vi "BuildingSingleImageGreyLevelDataBase.vi"(6 "Running Index":i32, 8 "error in (no error)":errorcluster, 9 "ConfDB":T1={"NumberOfImages"=0, "NoImages2SaveAroundFreeze"=0, "Path"=path "", "NameOfPartialFile"="", "StartIndex"=0, "NumberOfStdTol"=0, "Detla t (sec)"=2, "Number of images for baseline"=10, "Temperature File Name"="", "Score"=15.0, "Index number of Files"=[], "End Index"=2187, "Temperature Array"=[], "TStartIndex"=2187}, 10 "Droplet Bounding Box":cluster{"x":sgl, "y":sgl}[][](array[cluster]), 11 "Image Ref In":T2) -> (0 "error out":errorcluster, 1 "Difference in Grey Level":dbl[](array[numeric]), 2 "GreyLevelArray":dbl[](array[numeric]))   [LabVIEW 2013]
doc: "Go over all images and retrieve Grey level of each drop and the difference between the i+1 and i image"
uses:
  <vilib>/vision/Image Controls.llb/IMAQ Image.ctl
  DB/ConfDB.ctl
  DB/DbEnum.ctl
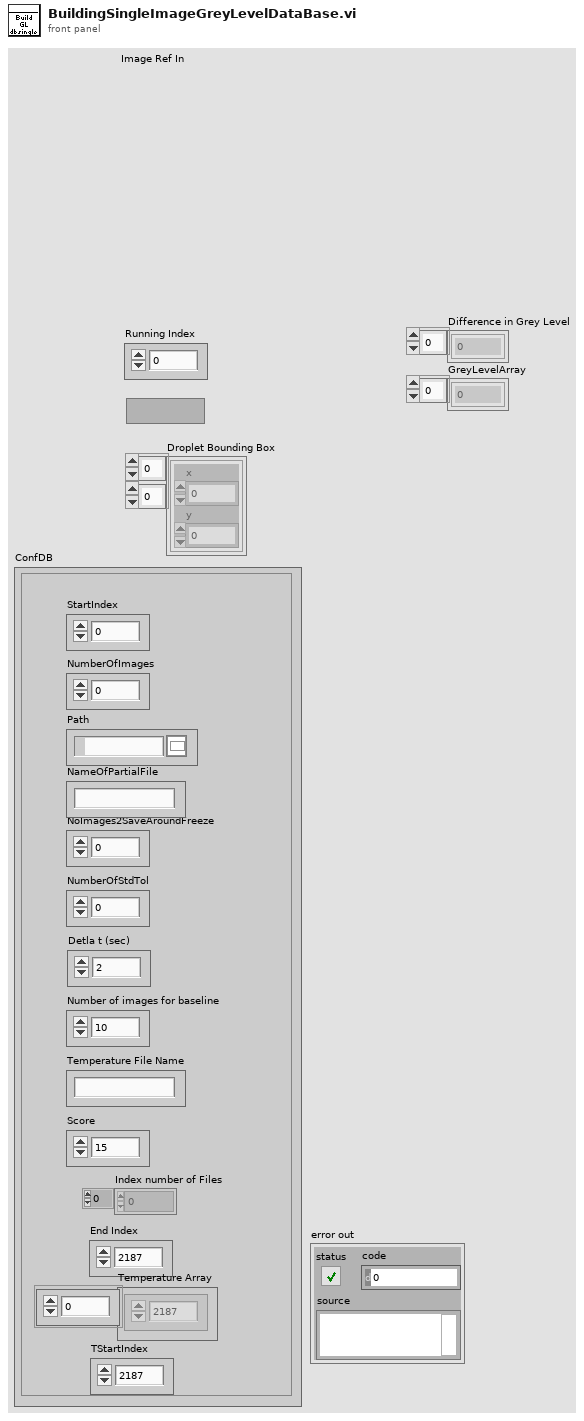
[diagram p1: front panel]
types:
  T1 = typedef "ConfDB.ctl" = cluster{"NumberOfImages":i32, "NoImages2SaveAroundFreeze":i32, "Path":path, "NameOfPartialFile":string, "StartIndex":i32, "NumberOfStdTol":i32, "Detla t (sec)":i32, "Number of images for baseline":i32, "Temperature File Name":string, "Score":dbl, "Index number of Files":i32[], "End Index":i32, "Temperature Array":dbl[], "TStartIndex":i32}
  T2 = typedef "IMAQ Image.ctl" = refnum<image>
  T3 = typedef "DbEnum.ctl" = enum16{"Write DropletDB", "Init", "Insert Detection Result Data", "Insert Grey Level Result", "Insert Baseline Results", "AddFreezeImagesAtCertainDroplet", "UpdateIncludeDroplet", "Insert Freeze Analysis Results", "GetDropDB", "GetNoFreezedDroplets", "GetGreyLevelAndDiff", "GetGreyLevelatIndexTime", "GetDropletsBoundingBox"}
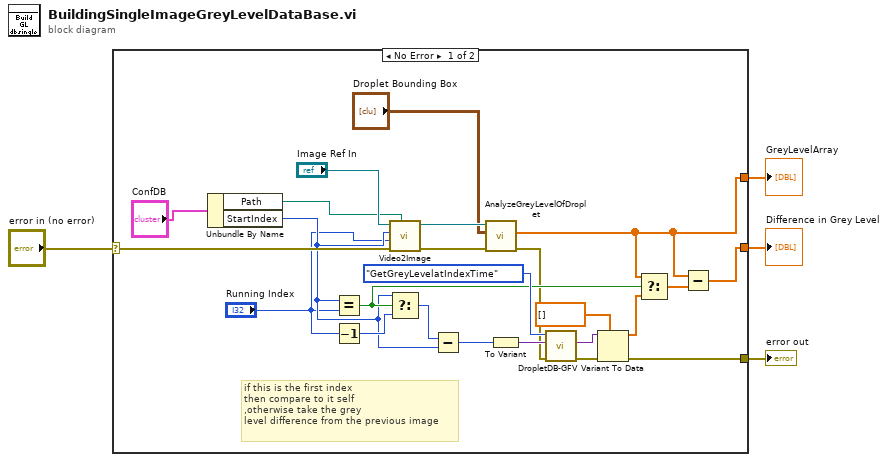
[diagram p0: block diagram]
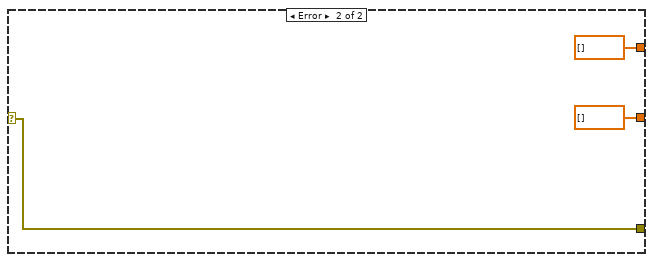
[diagram p2: hidden frame]
diagram:
  n1 = case shown="No Error" "error in (no error)" {
    selector: "error in (no error)" -> [w9 w31]
    tunnel: [w10 w31] -> w3
    tunnel: [w23 dbl[] []] -> w2
    tunnel: [w14 dbl[] [] ("GreyLevelArray")] -> w1
    frame No Error {
      # "if this is the first index\nthen compare to it self\n,otherwise take the grey\nlevel difference from the previous image"
      n2 = Unbundle By Name("ConfDB") -> ("Path"=w8:path, "StartIndex"=w7:i32)
      n3 = Equal?(x=w7, y="Running Index") -> (x = y?=w15:bool)
      n4 = Decrement(x="Running Index") -> (x-1=w24:i32)
      n5 = call "Video2Image.vi"("AVI File Path"=w8, "error in (no error)"=w9, "Running Index"="Running Index", "Start Index"=w7, "Image In"="Image Ref In") -> ("error out"=w11:errorcluster, "Image Out"=w26:T2)  [unwired: 5 in]
      n6 = Select(t=w7, s=w15, f=w24) -> (s? t:f=w18:i32)
      n7 = Subtract(x=w18, y=w7) -> (x-y=w16:i32)
      n8 = call "AnalyzeGreyLevelOfDroplet.vi"("error in (no error)"=w11, "Bounding Box"="Droplet Bounding Box", "Image In"=w26) -> ("error out"=w5:errorcluster, "GreyLevelArray"=w14:dbl[])  [unwired: 6 in, 1 out]
      n9 = To Variant(anything=w16) -> (Variant=w19:variant)
      n10 = call "DropletDB-GFV.vi"("error in (no error)"=w5, "Data in"=w19, "Command In"=DbEnum."GetGreyLevelatIndexTime") -> ("error out"=w21:errorcluster, "Data out"=w20:variant)  [unwired: 7 in]
      n11 = Variant To Data(error in=w21, type=dbl[] [] ("GreyLevelArray"), Variant=w20) -> (data=w13:dbl[], error out=w10:errorcluster)
      n12 = Select(t=w14, s=w15, f=w13) -> (s? t:f=w12:dbl[])
      n13 = Subtract(x=w14, y=w12) -> (x-y=w23:dbl[])
    }
    frame Error {
    }
  }
  "error out" <- w3
  "Difference in Grey Level" <- w2
  "GreyLevelArray" <- w1
